vi "ShellExec Master.vi"(4 "show":i32(ring)=1 items=["SW_HIDE", "SW_SHOWNORMAL", "SW_SHOWMINIMIZED"], 5 "operation":enum16{"open", "print"}(ring)=enum."print", 6 "default directory":path, 7 "command line parameters":string, 8 "error in (no error)":errorcluster, 11 "path to file":path) -> (0 "error out":errorcluster)   [LabVIEW 2023, in "Winevent.lvlib"]
doc: "This VI allows the user to either open or print a file as if it were selected from File Manager. Note that files whose extensions are not associated with an application will not be opened or printed.\n\nIf the VI is told to print a file, but the application that opens the file may not print a file, as dictated in the registration file, an error of -1027 is returned."
uses:
  Winevent.lvlib
  SHELL32.DLL
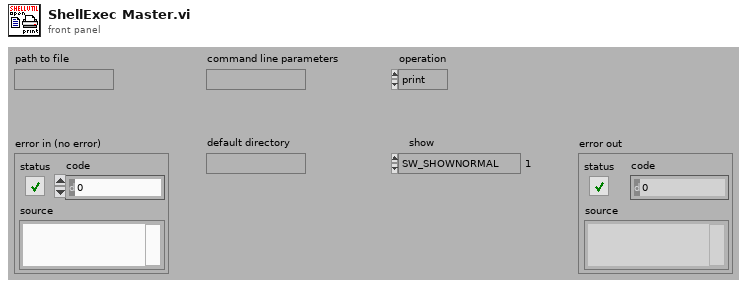
[diagram p1: front panel]
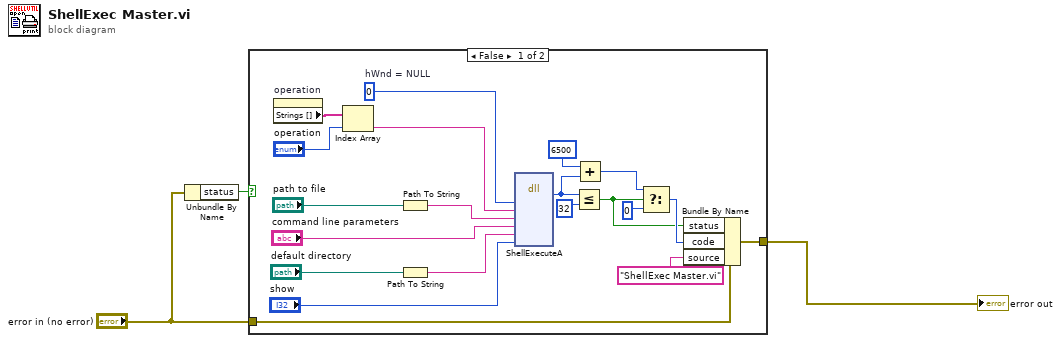
[diagram p0: block diagram]
diagram:
  n1 = Unbundle By Name("error in (no error)") -> ("status"=w3:bool)
  n2 = case shown="False" w3 {
    tunnel: "error in (no error)" -> [w6 w24]
    tunnel: [w5 w24] -> w2
    frame False {
      w23 = u32 0  # hWnd = NULL
      n3 = property on="operation" class="Enum (strict)"() -> ("Strings []"=w16:string[])  [unwired: 2 in, 2 out]
      n4 = Index Array(array=w16, index="operation") -> (element=w22:string)
      n5 = Path To String(path="path to file") -> (string=w21:string)
      n6 = Path To String(path="default directory") -> (string=w19:string)
      n7 = dll-call lib="SHELL32.DLL" fn="ShellExecuteA"("hWndParent"=w23, "lpszOp"=w22, "lpszFile"=w21, "lpszParams"="command line parameters", "lpszDir"=w19, "fsShowCmd"="show") -> ("hInstance"=w10:u32)  [unwired: 8 in, 3 out]
      n8 = Less Or Equal?(x=w10, y=u16 32) -> (x <= y?=w7:bool)
      n9 = Add(x=6500, y=w10) -> (x+y=w4:u32)
      n10 = Select(t=w4, s=w7, f=0) -> (s? t:f=w8:u32)
      n11 = Bundle By Name(cluster=w6, "status"=w7, "code"=w8, "source"="ShellExec Master.vi") -> (w5:errorcluster)
    }
    frame True {
    }
  }
  "error out" <- w2
